vi "H5Olink.vi"(4 "lcpl_id":T1, 6 "lapl_id":T1, 8 "error in (no error)":errorcluster, 9 "Object Ref":T1, 10 "Link Name":string, 11 "Location Ref":T1) -> (0 "error out":errorcluster, 3 "Location Ref out":T1)   [LabVIEW 2017]
doc: "Creates a hard link to an object in an HDF5 file."
uses:
  <vilib>/UPVI/lvhdf5/library.llb/HDF5 Ref.ctl
  <vilib>/UPVI/lvhdf5/hdf5.dll
panel:
  # "LVHDF5 Toolkit\nCopyright (c) 2005-2013 by Jason D. Sommerville\nCopyright (c) 2014-2015 by UPVI, LLC.\n\nThis use and distribution of this file is governed by the terms found in \nLICENSE.txt distributed with this toolkit and installed at\n <user.lib>\\_lvhdf5\\LICENSE.txt"
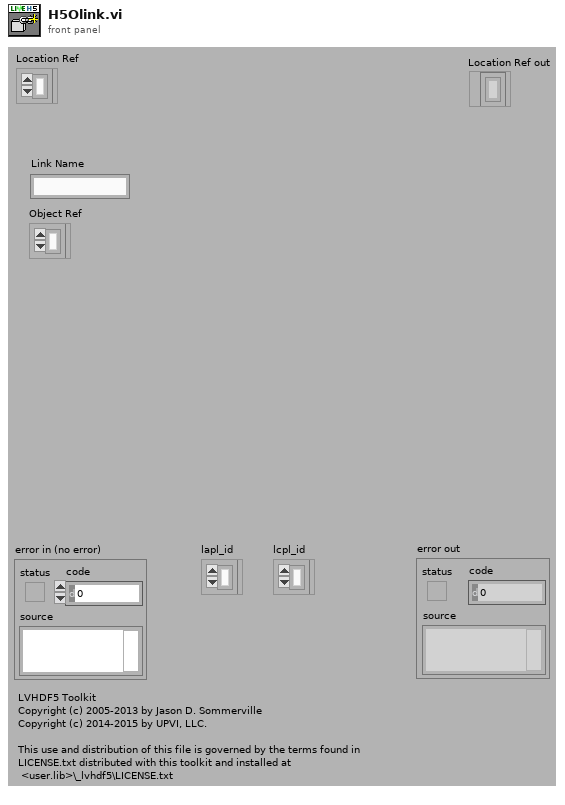
[diagram p1: front panel]
types:
  T1 = typedef "HDF5 Ref.ctl" = refnum<k1>
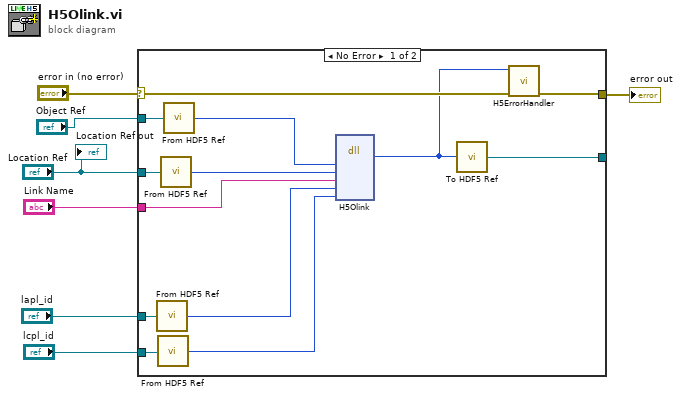
[diagram p0: block diagram]
diagram:
  n1 = case shown="No Error" "error in (no error)" {
    selector: "error in (no error)" -> [w20 w21]
    tunnel: [w19 w21] -> w6
    tunnel: "Location Ref" -> [w18 _]
    tunnel: "lapl_id" -> [w17 _]
    tunnel: [w14 _] -> _
    tunnel: "Object Ref" -> [w12 _]
    tunnel: "lcpl_id" -> [w10 _]
    tunnel: "Link Name" -> [w8 _]
    frame No Error {
      n2 = call <vilib>:"From HDF5 Ref.vi"("HDF5 Ref"=w17) -> ("I32"=w16:i32)
      n3 = call <vilib>:"From HDF5 Ref.vi"("HDF5 Ref"=w10) -> ("I32"=w9:i32)
      n4 = call <vilib>:"From HDF5 Ref.vi"("HDF5 Ref"=w18) -> ("I32"=w13:i32)
      n5 = call <vilib>:"From HDF5 Ref.vi"("HDF5 Ref"=w12) -> ("I32"=w11:i32)
      n6 = dll-call lib="C:/Program Files/National Instruments/LabVIEW 2017/vi.lib/UPVI/lvhdf5/hdf5.dll" fn="H5Olink" label="H5Oopen_by_index"("object_id"=w11, "new_loc_id"=w13, "name"=w8, "lapl_id"=w16, "lcpl_id"=w9) -> ("return type"=w15:i32)  [unwired: 8 in, 2 out]
      n7 = call <vilib>:"To HDF5 Ref.vi"("I32"=w15) -> ("HDF5 Ref"=w14:T1)
      n8 = call <vilib>:"H5ErrorHandler.vi"("error in (no error)"=w20, "herr_t"=w15) -> ("error out"=w19:errorcluster)  [unwired: 3 in, 4 out]
    }
    frame Error {
    }
  }
  "error out" <- w6
  "Location Ref out" <- "Location Ref"
